vi "Match Pattern.vi"(8 "Pattern":string, 9 "String in":string) -> (0 "String out":string, 1 "Match?":bool)   [LabVIEW 2017, in "XTree.xctl"]
uses:
  <vilib>/addons/_NIFileIO/XTree/XTree.xctl
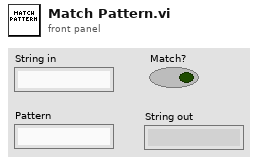
[diagram p1: front panel]
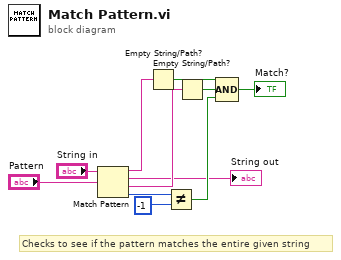
[diagram p0: block diagram]
diagram:
  # "Checks to see if the pattern matches the entire given string"
  n1 = Match Pattern(string="String in", regular expression="Pattern") -> (before substring=w8:string, match substring=→"String out":string, after substring=w9:string, offset past match=w6:i32)  [unwired: 1 in]
  n2 = Empty String/Path?(string/path=w8) -> (empty?=w10:bool)
  n3 = Not Equal?(x=w6, y=-1) -> (x != y?=w5:bool)
  n4 = Empty String/Path?(string/path=w9) -> (empty?=w11:bool)
  n5 = Compound Arithmetic op=AND(w10, w11, w5) -> (→"Match?":bool)
